vi "generate table.vi"(7 "table":T1, 8 "error in":errorcluster, 10 "engine configuration":refnum<class "engine configuration.lvclass">, 11 "tag bus configurable plugin module configuration":refnum<class "Tagbus PID Module configuration.lvclass">) -> (0 "error out":errorcluster)   [LabVIEW 2014, in "Tagbus PID Module editor node.lvclass"]
uses:
  Tagbus PID Module editor node.lvclass
  table reference.ctl
  module/configuration/Tagbus PID Module configuration.lvclass
  <vilib>/NI/Module Execution Interface/Engine Configuration/engine configuration.lvclass
  <vilib>/NI/Configuration Framework/serializable configuration/NISE_CEF_serializable configuration.lvclass/NISE_CEF_serializable configuration.ctl
  table line.ctl
  <vilib>/NI/Tag Bus Module Framework/channel/TBM channel.lvclass
  <vilib>/NI/Tag Bus/tag/read tag name.vi
  <vilib>/NI/Configuration Framework/serializable configuration/Read UID.vi
  <vilib>/Utility/LVClass/Get LV Class Name.vi
  <vilib>/NI/Configuration Framework/error generator/NISE_error generator.vi
  <vilib>/NI/Tag Bus/tag/tag descriptor.lvclass
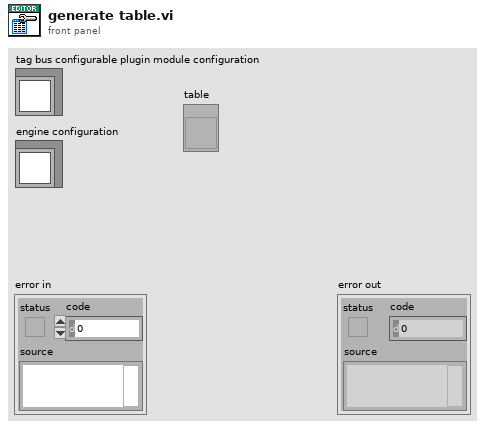
[diagram p1: front panel]
types:
  T1 = typedef "Tagbus PID Module editor node.lvclass/table reference.ctl" = refnum<vi>
  T2 = cluster{"ID":string, "Setpoint":refnum<class "TBM channel.lvclass">, "Process Variable":refnum<class "TBM channel.lvclass">, "Output":refnum<class "TBM channel.lvclass">, "PID gains":cluster{"proportional gain (Kc)":dbl, "integral time (Ti, min)":dbl, "derivative time (Td, min)":dbl}, "output range":cluster{"output high":dbl, "output low":dbl}}[]
  T3 = typedef "Tagbus PID Module editor node.lvclass/table line.ctl" = cluster{"ID":string, "Setpoint":refnum<class "TBM channel.lvclass">, "Process Variable":refnum<class "TBM channel.lvclass">, "Output":refnum<class "TBM channel.lvclass">, "PID gains":cluster{"proportional gain (Kc)":dbl, "integral time (Ti, min)":dbl, "derivative time (Td, min)":dbl}, "output range":cluster{"output high":dbl, "output low":dbl}}
  T4 = cluster{"proportional gain (Kc)":dbl, "integral time (Ti, min)":dbl, "derivative time (Td, min)":dbl}
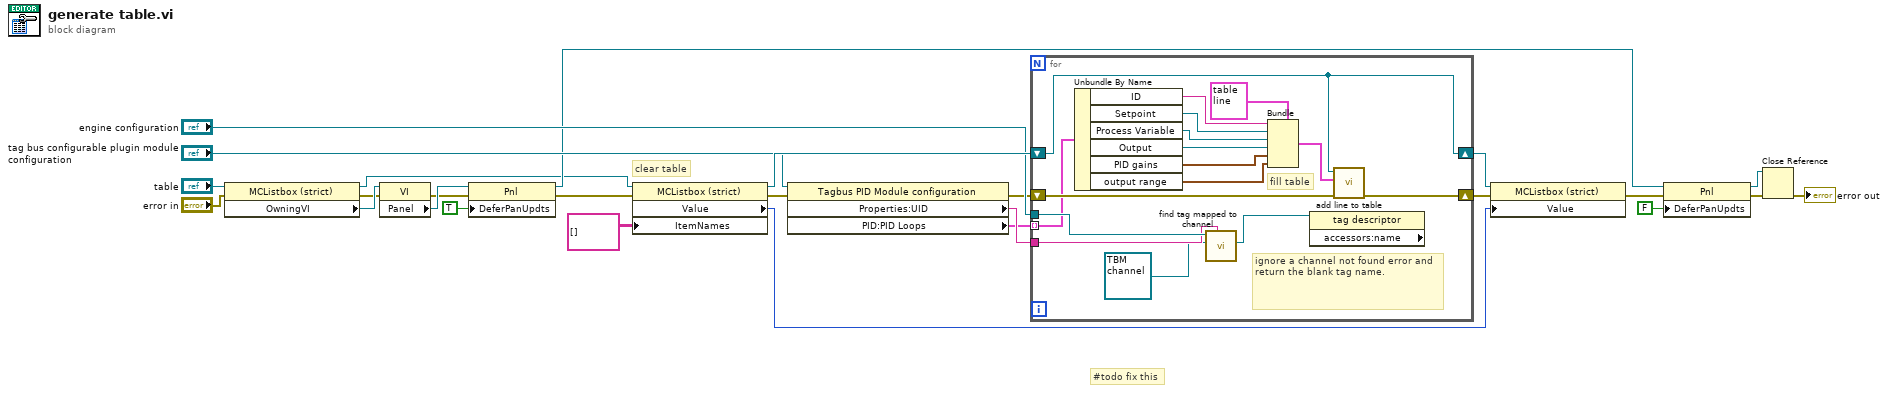
[diagram p0: block diagram]
diagram:
  # "#todo fix this"
  # "clear table"
  n1 = property class="MCListbox (strict)"(reference="table", error in="error in") -> (reference out=w7:T1, error out=w4:errorcluster, "OwningVI"=w5:refnum<vi>)
  n2 = property class="VI"(reference=w5, error in=w4) -> (error out=w13:errorcluster, "Panel"=w14:refnum<vi>)  [unwired: 1 out]
  n3 = property class="Pnl"(reference=w14, error in=w13, "DeferPanUpdts"=TRUE ("Defer Panel Updates")) -> (reference out=w10:refnum<vi>, error out=w12:errorcluster)
  n4 = property class="MCListbox (strict)"(reference=w7, error in=w12, "ItemNames"=string[][] [] ("Item Names")) -> (reference out=w25:T1, error out=w21:errorcluster, "Value"=w16:i32)
  n5 = property class="Tagbus PID Module configuration"(reference="tag bus configurable plugin module configuration", error in=w21) -> (error out=w20:errorcluster, "Properties:UID"=w22:string, "PID:PID Loops"=w1:T2)  [unwired: 1 out]
  n6 = for {
    shift-right: [w42] -> w17
    shift-left: w20 -> [w39]
    tunnel: "engine configuration" -> [w38]
    tunnel: w22 -> [w37]
    shift-right: [w35] -> w18
    shift-left: w25 -> [w35]
    tunnel: w1 -> [w34] mode=indexing
    # "ignore a channel not found error and return the blank tag name."
    # "fill table"
    n7 = Unbundle By Name(w34) -> ("ID"=w33:string, "Setpoint"=w32:refnum<class "TBM channel.lvclass">, "Process Variable"=w31:refnum<class "TBM channel.lvclass">, "Output"=w30:refnum<class "TBM channel.lvclass">, "PID gains"=w29:T4, "output range"=w28:cluster{"output high":dbl, "output low":dbl})
    n8 = call <vilib>:"find tag mapped to channel.vi"("owner"=w37, "channel"=refnum<class "TBM channel.lvclass"> refnum, "engine configuration in"=w38) -> ("tag"=w36:refnum<class "tag descriptor.lvclass">)  [unwired: 6 in, 2 out]
    n9 = Bundle(cluster=T3 {"ID"="", "Setpoint"=refnum, "Process Variable"=refnum, "Output"=refnum, "PID gains"={"proportional gain (Kc)"=1.0, "integral time (Ti, min)"=0.01, "derivative time (Td, min)"=0.0}, "output range"={"output high"=100.0, "output low"=-100.0}} ("line"), "ID"=w33, "Setpoint"=w32, "Process Variable"=w31, "Output"=w30, "PID gains"=w29, "output range"=w28) -> (w40:T3)
    n10 = property class="tag descriptor" props=["accessors:name"](reference=w36) -> ()  [unwired: 1 in, 3 out]
    n11 = call "add line to table.vi"("error in"=w39, "line"=w40, "operations table"=w35) -> ("error out"=w42:errorcluster)  [unwired: 8 in]
  }
  n12 = property class="MCListbox (strict)"(reference=w18, error in=w17, "Value"=w16) -> (error out=w9:errorcluster)  [unwired: 1 out]
  n13 = property class="Pnl"(reference=w10, error in=w9, "DeferPanUpdts"=FALSE ("Defer Panel Updates")) -> (reference out=w2:refnum<vi>, error out=w8:errorcluster)
  n14 = Close Reference(reference=w2, error in (no error)=w8) -> (error out=→"error out":errorcluster)
